vi "IBM4_Diff_Read.vi"   [LabVIEW 2021, in "IBM4.lvlib"]
doc: "Differntial Read from IBM4 (Binary or Voltage)\nThere are 5 different read options:\n1) Single binary/inteter reading\n2) Multiple binary/integer readings\n3) Single Voltage reading\n4) Multiple Voltage readings\n5) Average Voltage from multiple readings"
uses:
  <instrlib>/IBM4/IBM4.lvlib
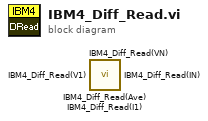
[diagram p0: block diagram]
diagram:
  n1 = call <instrlib>:"IBM4_Diff_Read(Ave).vi"() -> ()  [unwired: 9 in, 3 out]
  n2 = call <instrlib>:"IBM4_Diff_Read(VN).vi"() -> ()  [unwired: 9 in, 3 out]
  n3 = call <instrlib>:"IBM4_Diff_Read(V1).vi"() -> ()  [unwired: 9 in, 3 out]
  n4 = call <instrlib>:"IBM4_Diff_Read(IN).vi"() -> ()  [unwired: 9 in, 3 out]
  n5 = call <instrlib>:"IBM4_Diff_Read(I1).vi"() -> ()  [unwired: 9 in, 3 out]
